vi "Strings to Connections.vi"(8 "error in":errorcluster, 10 "connection strings":string[](array[string]), 11 "routing and faulting in":T1 format="%.0x") -> (0 "error out":errorcluster, 2 "connection list":T2[](array[typedef]), 3 "routing and faulting out":T1 format="%.0x")   [LabVIEW 2020, in "Routing and Faulting Scripting.lvlib"]
uses:
  Routing and Faulting Scripting.lvlib
  Shared/Connection.ctl
  <vilib>/NI VeriStand/Custom Device API/Custom Device Item Ref.ctl
  Shared/Routing and Faulting Shared.lvlib
  <vilib>/NI VeriStand/Custom Device API/Custom Device API.lvlib
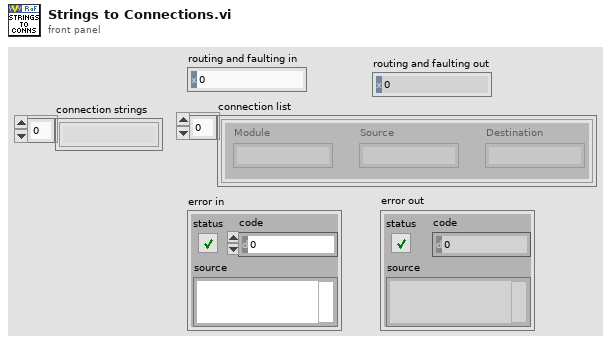
[diagram p1: front panel]
types:
  T1 = typedef "Custom Device API.lvlib/Custom Device Item Ref.ctl" = u64
  T2 = typedef "Routing and Faulting Shared.lvlib/Connection.ctl" = cluster{"Module":string, "Source":string, "Destination":string}
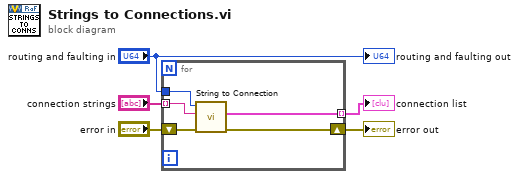
[diagram p0: block diagram]
diagram:
  n1 = for {
    tunnel: "connection strings" -> [w10] mode=indexing
    tunnel: "routing and faulting in" -> [w9]
    shift-right: [w7] -> w1
    shift-left: "error in" -> [w8]
    tunnel: [w6] -> w2 mode=indexing
    n2 = call "String to Connection.vi"("error in"=w8, "string"=w10, "routing and faulting in"=w9) -> ("error out"=w7:errorcluster, "connection"=w6:T2)  [unwired: 6 in, 1 out]
  }
  "connection list" <- w2
  "error out" <- w1
  "routing and faulting out" <- "routing and faulting in"
